vi "EngineeringGlobals.vi"() -> ()   [LabVIEW 2014]
panel:
  in  "Tab Control":enum32{"Flags", "Admin", "Files"}(tab)=enum."Admin"
  out "CloseServer":bool
  out "AutoTitle":bool=TRUE
  out "FocusMode":bool
  out "SocketOpen":bool
  out "TestImage":bool=TRUE
  out "UserWarnings":bool=TRUE
  out "DemoMode":bool
  out "RemoteFileEnable":bool
  out "ClearArray":bool=TRUE
  out "Sound":bool
  out "Prompt4Title":bool
  out "ReadTemps":bool
  out "AutoCamInit":bool=TRUE
  in  "ImageType":string="zero"
  in  "ImageTypes":string[](array[string])=["zero", "object", "flat", "dark", "ramp"]
  in  "ConnectionID 3":refnum<k5>
  in  "ClientHostName":string="lesser.itl.arizona.edu"
  in  "SystemModule":string="NONE"
  in  "ConnectionID 2":refnum<k5>
  in  "LastTitle":string
  in  "ClientHostIP":string="10.0.0.122"
  in  "Title":string="zero"
  in  "Version":string="06Jun08"
  in  "GlobalsList":string[](array[string])=["ServerName", "ServerPort", "Sound", "AutoCamInit", "Prompt4Header", "ImageHeaderTemplateFile", "FPposition", "FileServerPath", "SystemDir", "CloseServer", "SystemModule", "AutoTitle", "PythonPath", "EditorPath", "UserWarnings"]
  in  "ImageFormat":T1(ring)=enum."FITS"
  in  "ServerPort":i32=2402
  in  "ServerName":string="lesser"
  in  "ConnectionID":refnum<k5>
  in  "UpdaterRef":refnum<vi>
  in  "AzCamToolRef":refnum<vi>
  out "OS":i32=3
  in  "FPposition":string="5 794"
  in  "EditorPath":path=path "notepad.exe"
  in  "PythonPath":path=path "c:/azcam/StartPython.bat"
  in  "RootDir":path=path "C:/AzCam/source/AzCamTool"
  in  "Filename":string="!c:/data/test.fits"
  in  "SoundReadout":path=path "C:/azcam/systems/itl/detchar/snd_readout_finished.wav"
  in  "SoundExposure":path=path "C:/azcam/systems/itl/detchar/snd_exposure_finished.wav"
  in  "ParFile":path=path "C:/data/Defaults/AzCamToolDefaults.ini"
  in  "SystemDir":path=path "C:/azcam/systems/itl/detchar"
  in  "ImageHeaderTemplateFile":path=path "C:/AzCam/systems/ITL/DetChar/FitsTemplate_DetChar.txt"
  in  "FileServer Path":path
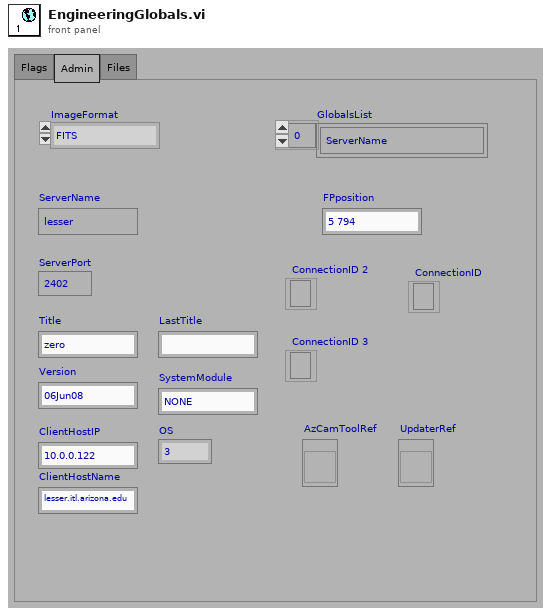
[diagram p1: front panel]
types:
  T1 = enum16{"unused", "FITS", "Binary", "Extended FITS"}
diagram:
